vi "Metronome_atchaj.vi"() -> ()   [LabVIEW 2015]
panel:
  in  "stop":bool
  in  "Numeric":dbl
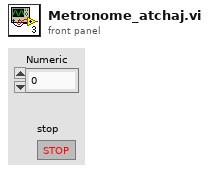
[diagram p1: front panel]
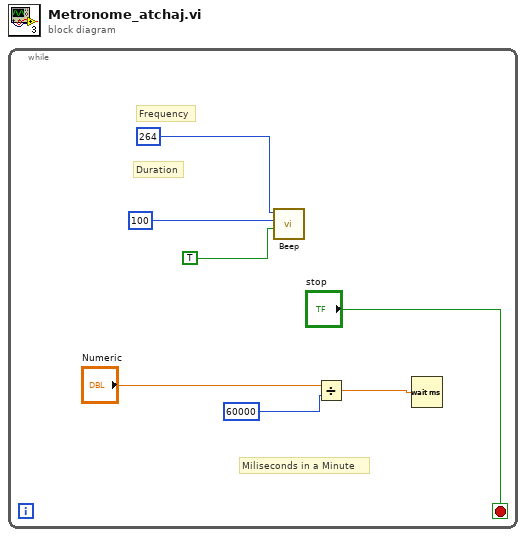
[diagram p0: block diagram]
diagram:
  n1 = while {
    stop <- "stop" stop-if-true
    # "Duration"
    # "Frequency"
    # "Miliseconds in a Minute"
    n2 = call <vilib>:"Beep.vi"("use system alert? (T)"=TRUE, "duration (msec)"=u32 100, "frequency (Hz)"=u32 264) -> ()  [unwired: 9 in]
    n3 = Divide(x="Numeric", y=60000) -> (x/y=w2:dbl)
    n4 = Wait (ms)(milliseconds to wait=w2) -> ()  [unwired: 1 out]
  }
